vi "NML Data Acquisition.vi"() -> ()   [LabVIEW 2025]
doc: "Author: Scott Hannahs <sth@magnet.fsu.edu>\n\nThis software is licensed for use under the “MIT License\"\nCopyright (c) 2025 Scott Hannahs, sth@sth@magnet.sthnet.net\n\nPermission is hereby granted, free of charge, to any person obtaining a copy of this software and associated documentation files (the \"Software\"), to deal in the Software without restriction, including without limitation the rights to use, copy, modify, merge, publish, distribute, sublicense, and/or sell copies of the Software, and to permit persons to whom the Software is furnished to do so, subject to the following conditions: The above copyright notice and this permission notice shall be included in all copies or substantial portions of the Software.\n\nTHE SOFTWARE IS PROVIDED \"AS IS\", WITHOUT WARRANTY OF ANY KIND, EXPRESS OR IMPLIED, INCLUDING BUT NOT LIMITED TO THE WARRANTIES OF MERCHANTABILITY, FITNESS FOR A PARTICULAR PURPOSE AND NONINFRINGEMENT. IN NO EVENT SHALL THE AUTHORS OR COPYRIGHT HOLDERS BE LIABLE FOR ANY CLAIM, DAMAGES OR OTHER LIABILITY, WHETHER IN AN ACTION OF CONTRACT, TORT OR OTHERWISE, ARISING FROM, OUT OF OR IN CONNECTION WITH THE SOFTWARE OR THE USE OR OTHER DEALINGS IN THE SOFTWARE."
uses:
  <userlib>/_OpenG.lib/file/file.llb/openg_file.lvlib
panel:
  in  "Launch Old":bool
  in  "Launch New":bool
  # "Please report suggestions, problems or issues to Scott Hannahs <sth@magnet.fsu.edu>"
  # "Launch the Old NML Data Acquisition sytem.\nUse this version for instruments still unsupported by the new version."
  # "Launch the New NML Data Acquisition sytem.\nThis improved version easier to configure version can access temperature  \ncontrollers, voltmeters, capacitance bridges, \nand SRS and Signal Recovery lockin amplifiers"
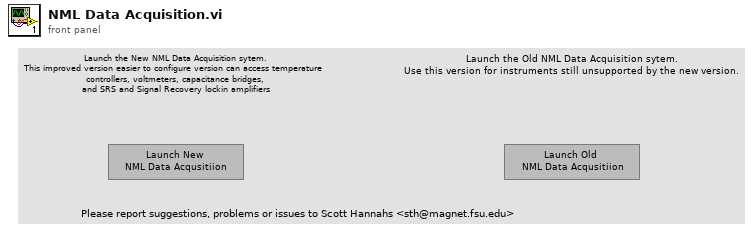
[diagram p1: front panel]
types:
  T1 = enum32{"Invalid", "Standard", "Closed", "Hidden", "Minimized", "Maximized"}
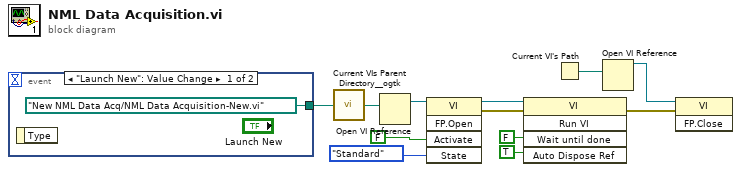
[diagram p0: block diagram]
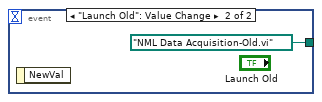
[diagram p2: hidden frame]
diagram:
  n1 = event shown="[0] \"Launch New\": Value Change" {
    selector: _ -> [_ _]
    dyn-events: _ -> [_ _]
    timeout: _ -> [_ _]
    tunnel: [path "New NML Data Acq/NML Data Acquisition-New.vi" path "NML Data Acquisition-Old.vi"] -> w6
    event "Launch New": Value Change {
      n2 = event-data() -> ()  [unwired: 1 in, 1 out]
    }
    event "Launch Old": Value Change {
      n3 = event-data() -> ()  [unwired: 1 in, 1 out]
    }
  }
  n4 = call <userlib>:"Current VIs Parent Directory__ogtk.vi"("Relative path (.)"=w6) -> ("Parent Directory (+ Relative)"=w7:path)  [unwired: 4 in]
  n5 = Open VI Reference(vi path=w7) -> (vi reference=w8:refnum<vi>)  [unwired: 5 in, 1 out]
  n6 = invoke class="VI" method="FP.Open"(reference=w8, "Activate"=FALSE ("Activate?"), "State"=T1."Standard") -> (reference out=w4:refnum<vi>, error out=w5:errorcluster)  [unwired: 2 in, 3 out]
  n7 = invoke class="VI" method="Run VI"(reference=w4, error in=w5, "Wait until done"=FALSE ("Wait Until Done"), "Auto Dispose Ref"=TRUE ("Auto Dispose Reference")) -> (error out=w1:errorcluster)  [unwired: 1 in, 4 out]
  n8 = Current VI's Path() -> (path=w10:path)
  n9 = Open VI Reference(vi path=w10) -> (vi reference=w9:refnum<vi>)  [unwired: 5 in, 1 out]
  n10 = invoke class="VI" method="FP.Close"(reference=w9, error in=w1) -> ()  [unwired: 1 in, 3 out]
